vi "TLB Native Dynamic Events ver 0.08.vi"() -> ()   [LabVIEW 2018]
uses:
  Labview Training Phase 2/Enum Controls/States for Action Engine.ctl
  Type def/TLB event states.ctl
  Type def/TLB MHL States.ctl
  <vilib>/Studica/Studica Toolkit/Background/I2C Channel.ctl
  <vilib>/Studica/Studica Toolkit/NavX/NavX.lvlib
  <vilib>/myRIO/Common/Instrument Driver Framework/myRIO v1.0/AI/typedefs/AI Channels Enum.ctl
  <vilib>/myRIO/Common/Instrument Driver Framework/myRIO v1.0/AI/typedefs/AI Channels List.ctl
  Type def/Type def.ctl
  <vilib>/Studica/Studica Blackhawk/Blackhawk.lvlib
  <vilib>/Studica/Studica Toolkit/Background/Mxp Selection.ctl
  <vilib>/Studica/Studica Toolkit/Background/DIO Channel.ctl
  <vilib>/NI_Real-Time Target Support.lvlib
  <vilib>/ptbypt/NI_PtbyPt.lvlib
  <vilib>/addons/control/pid/NI_PID_pid.lvlib
  <vilib>/addons/control/pid/pid.llb/PID (DBL).vi
  Underlying VI's/Webcam FGV Low level ver/State control.ctl
  <vilib>/userdefined/High Color/IMAQdx.ctl
panel:
  out "Manual Zero Yaw":bool
  out "Displacement":T1
  out "Fused Heading":dbl
  in  "error in (no error)":errorcluster
  in  "RED LED State":enum16{"OFF", "ON", "BLINK"}(ring)
  in  "GREEN LED State":enum16{"OFF", "ON", "BLINK"}(ring)
  in  "Red LED":bool
  in  "Green LED":bool
  in  "NavX Zero Yaw":bool
  out "Input state":i8
  out "Waveform Chart 2":dbl(graph)
  out "Waveform Chart":dbl(graph)
  in  "STOP":bool
  out "DIO 0":bool
  out "DIO 1":bool
  out "Limit Switch Array":bool[](array[boolean])
  out "error out":errorcluster
  out "L/R average":fxp<+,64,64>
  out "Right Ultrasonic":fxp<+,64,16>
  out "Left Ultrasonic":fxp<+,64,16>
  out "Right IR Sensor":dbl
  out "Left IR Sensor":dbl
  out "Object detection count":T2
  out "Camera error":errorcluster
  in  "Servo Angle":u8(slide) scale=0.0..180.0
  in  "On/Off":bool
  out "Error":errorcluster
  out "element":T3
  out "Action Queue Items":i32
  out "State Logic Queue Items":i32
  out "Action Queues items":string[](array[string])=["Hardware reset", "Software reset", ""]
  out "State logic":T4=enum."Task 2"
  out "Action State":string
  out "Yaw":dbl
  # "TLB FRAMEWORK STATUS"
  # "Camera Status Loop"
  # "Test Programme written by Calvin Loke    Dated: 28 Aug 2019\nTest Programme revised by Dr Alex See   Dated 30 Aug 2019\n\nProgramme version:   TLB Native Dynamic Events ver 0.04b.vi"
  # "Problems now:\nYaw does not work when code is in last state mode\nSlow acceleration due to loop rate?"
  # "Motor Control Loop"
  # "NAVX Control Loop"
  # "Blackhawk status"
  # "Sensor data"
  # "System Health Status Update"
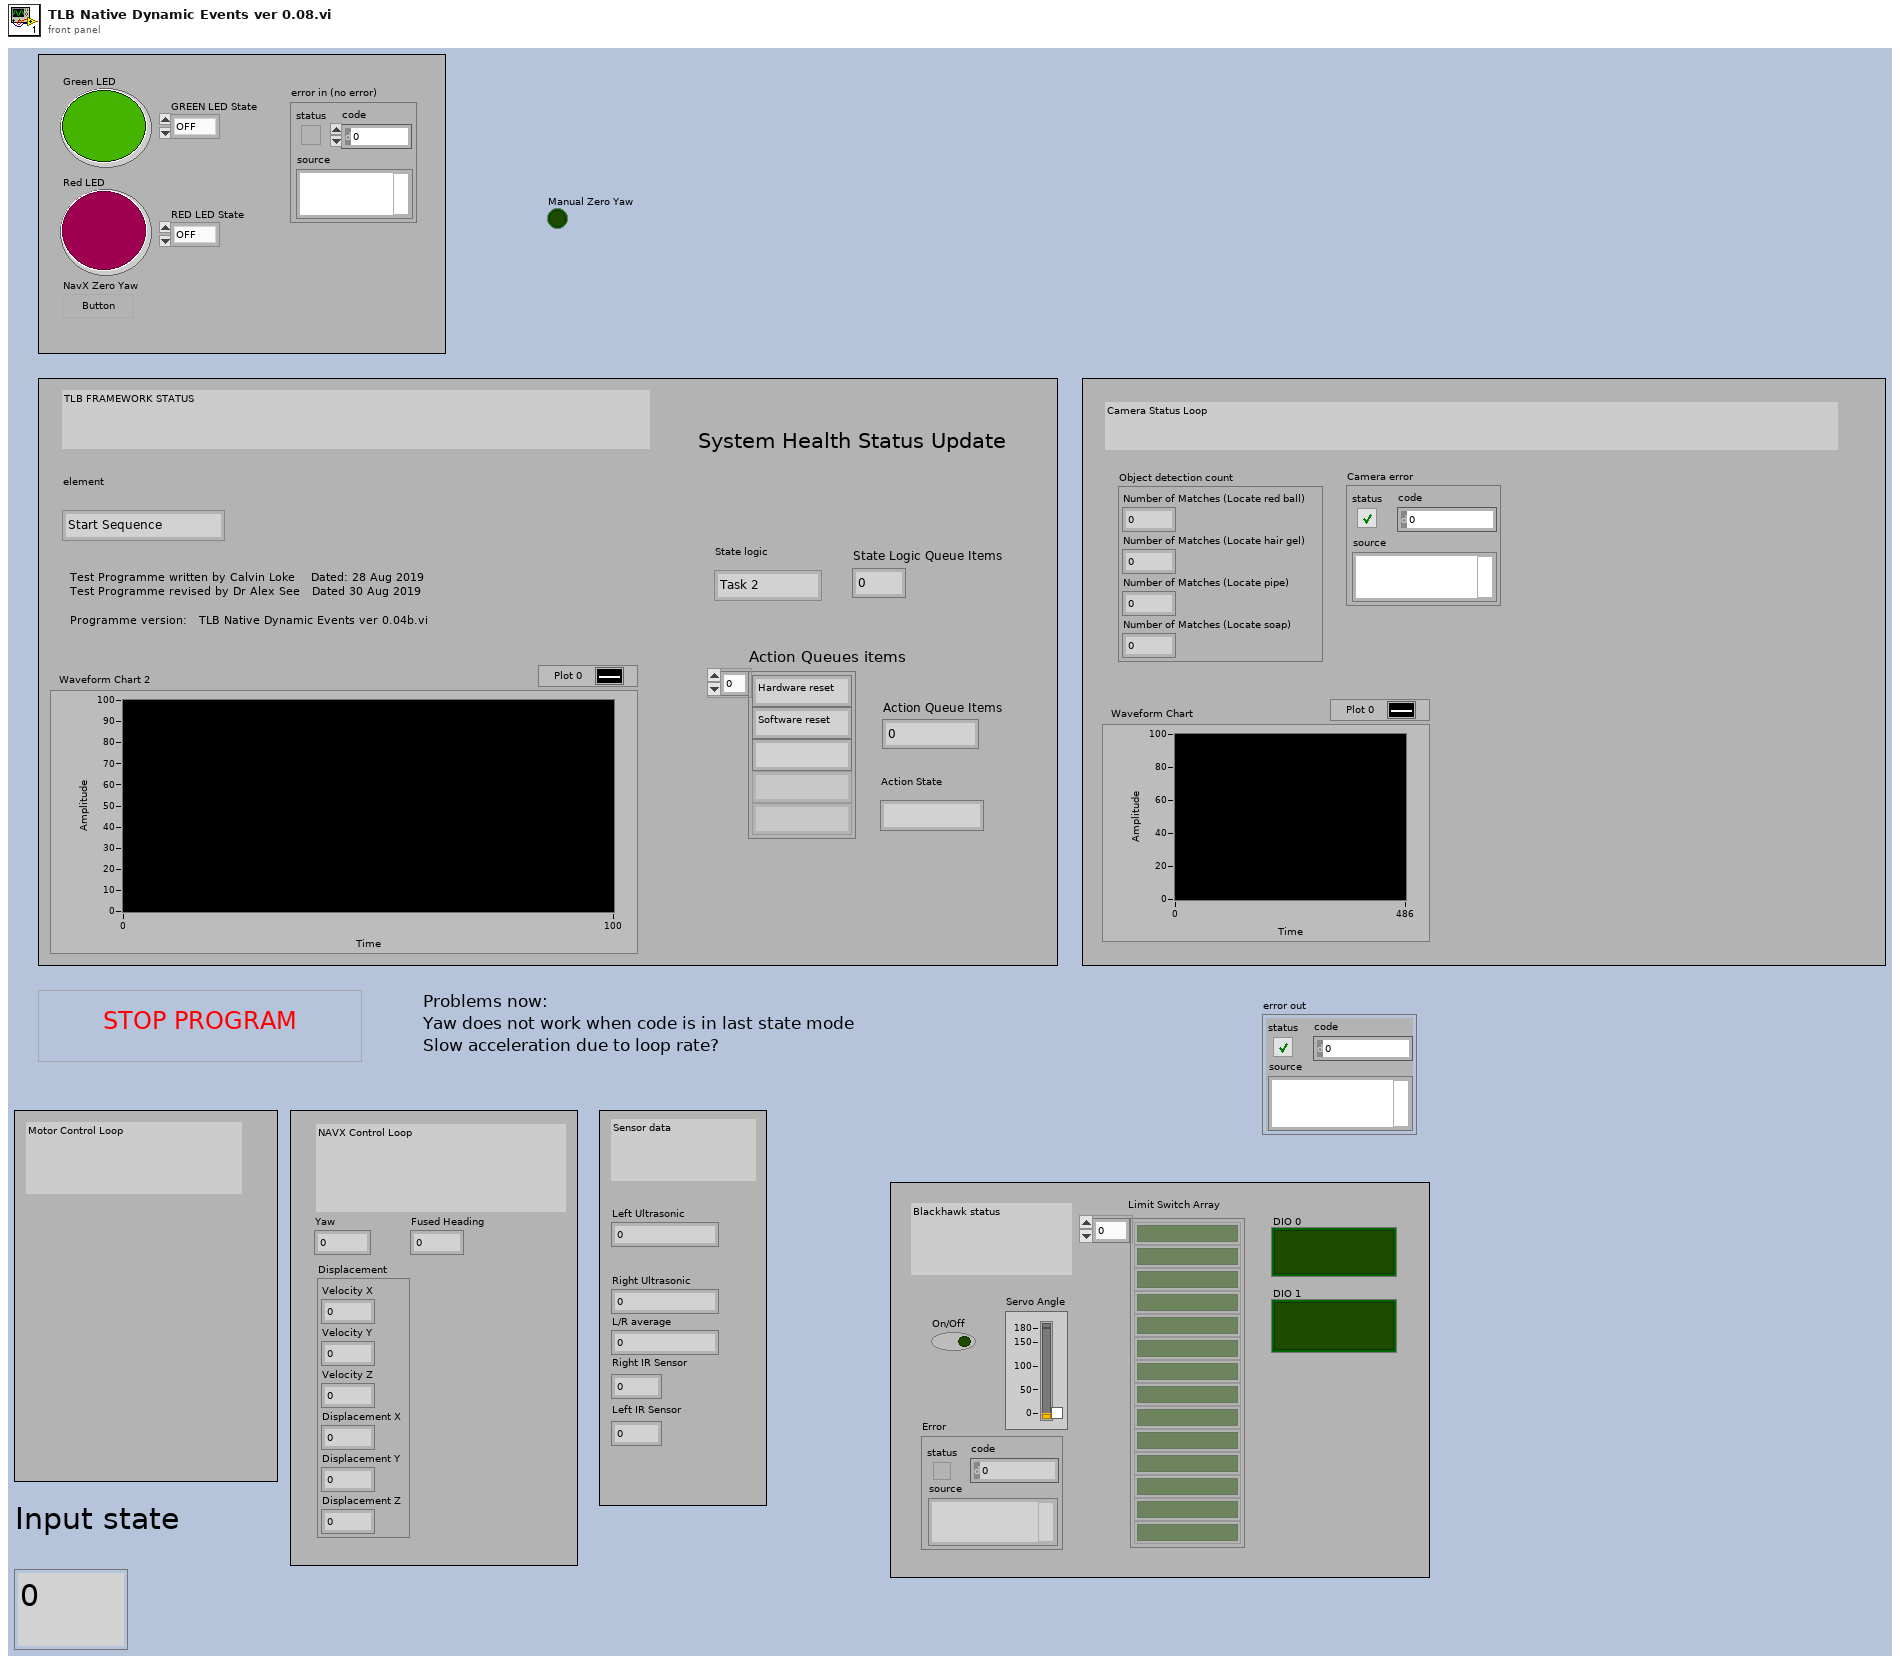
[diagram p1: front panel]
types:
  T1 = cluster{"Velocity X":dbl, "Velocity Y":dbl, "Velocity Z":dbl, "Displacement X":dbl, "Displacement Y":dbl, "Displacement Z":dbl}
  T2 = cluster{"Number of Matches (Locate red ball)":i32, "Number of Matches (Locate hair gel)":i32, "Number of Matches (Locate pipe)":i32, "Number of Matches (Locate soap)":i32}
  T3 = typedef "TLB event states.ctl" = enum16{"Start Sequence", "Exit", "Start Task 1", "Start Task 2", "Start Task 3", "Start Task 4", "Camera vision", "Wall follow mode", "Idle", "Start Drive Straight"}
  T4 = typedef "TLB MHL States.ctl" = enum16{"None", "Startup", "Idle", "Processing", "Shutdown", "Reset", "Task 1", "Task 2", "Task 3", "Task 4", "Task 4a", "Task 4b", "Task 4c", "Task 4d", "Task 4e", "Task 4f", "Task 4g", "Task 4h", "Acquire image", "Wall follow mode", "Autodrive", "Autodrive a"}
  T5 = typedef "States for Action Engine.ctl" = enum16{"Initialize", "Write", "Read"}
  T6 = typedef "DIO Channel.ctl" = enum16{"Not Connected", "A/DIO1", "A/DIO2", "A/DIO3", "A/DIO4", "A/DIO5", "A/DIO6", "A/DIO7", "A/DIO13", "B/DIO1", "B/DIO2", "B/DIO3", "B/DIO4", "B/DIO5", "B/DIO6", "B/DIO7", "B/DIO13", "C/DIO0", "C/DIO1", "C/DIO2", "C/DIO3", "C/DIO4", "C/DIO5", "C/DIO6", "C/DIO7"}
  T7 = typedef "Type def.ctl" = cluster{"Front Ultrasonic Obstruct":bool, "Left Ultrasonic Obstruct":bool, "Right Ultrasonic Obstruct ":bool}
  T8 = typedef "I2C Channel.ctl" = enum16{"Not Connected", "A", "B"}
  T9 = typedef "TLB MHL States.ctl" = enum16{"None", "Startup", "Idle", "Processing", "Shutdown", "Reset", "Task 1", "Task 2", "Task 3", "Task 4", "Task 4a", "Task 4b", "Task 4c", "Task 4d", "Task 4e", "Task 4f", "Task 4g", "Task 4h", "Acquire image", "Wall follow mode", "Drive Straight"}
  T10 = enum16{"LAST STATE", "STOP", "FORWARD", "BACKWARD", "LEFT", "RIGHT", "RCW", "ACW", "INIT", "RESET ENCODERS"}
  T11 = cluster{"proportional gain (Kc)":dbl, "integral time (Ti, min)":dbl, "derivative time (Td, min)":dbl}
  T12 = typedef "State control.ctl" = enum16{"Initialise", "Start camera", "Continuous Acquisition ", "Stop camera", "Dispose all"}
  T13 = typedef "IMAQdx.ctl" = refnum<k21>
  T14 = typedef "Mxp Selection.ctl" = enum16{"MXP A", "MXP B"}
  T15 = enum16{"DISTANCE READ", "STOP", "FORWARD", "BACKWARD", "LEFT", "RIGHT", "RCW", "ACW", "INIT", "RESET ENCODERS"}
  T16 = typedef "AI Channels List.ctl" = T17[]
  T17 = typedef "AI Channels Enum.ctl" = enum16{"Not Connected", "AudioIn/Left", "AudioIn/Right", "C/AI0", "C/AI1", "A/AI0", "A/AI1", "A/AI2", "A/AI3", "A/AI4", "A/AI5", "A/AI6", "A/AI7", "B/AI0", "B/AI1", "B/AI2", "B/AI3", "B/AI4", "B/AI5", "B/AI6", "B/AI7", "AI/AI0", "AI/AI1", "AI/AI2", "AI/AI3", "A/AI0 (DIFF)", "A/AI1 (DIFF)", "A/AI2 (DIFF)", "A/AI3 (DIFF)", "B/AI0 (DIFF)", "B/AI1 (DIFF)", "B/AI2 (DIFF)", "B/AI3 (DIFF)"}
  T18 = cluster{"DIO Channel":T6, "FPGA VI Reference Out":refnum<k20>}
  T19 = typedef "Analog Scaling Constants List.ctl" = T20[]
  T20 = typedef "Analog Scaling Constants.ctl" = cluster{"LSB Weight (Volts)":dbl, "Offset (Volts)":dbl, "Signed?":bool}
  T21 = cluster{"Scale Constants Array":T19, "FPGA Reference Out":refnum<k20>, "AI Channel":T16}
  T22 = cluster{"I2C Channel":T8, "FPGA VI Reference Out":refnum<k20>}
  T23 = typedef "NI_Real-Time Target Support.lvlib/RT CPU Load.ctl" = cluster{"Total (%)":dbl, "Time Critical (%)":dbl, "Timed Structures (%)":dbl, "High (%)":dbl, "Above Normal (%)":dbl, "Normal (%)":dbl, "Background (%)":dbl, "Idle (%)":dbl, "ISR (%)":dbl}
  T24 = cluster{"CPU loads[0]":T23, "CPU loads[1]":T23, "CPU loads[2]":T23, "CPU loads[3]":T23, "CPU loads[4]":T23, "CPU loads[5]":T23, "CPU loads[6]":T23, "CPU loads[7]":T23, "CPU loads[8]":T23}
  T25 = cluster{"I2C Ref Out":cluster{"I2C Channel":T8, "FPGA VI Reference Out":refnum<k20>}, "Connected":bool, "Slave Address (7-bit)":u8, "Registry":u8[]}
  T26 = cluster{"Yaw":dbl, "Roll":dbl, "Pitch":dbl, "Heading":dbl, "Fused Heading":dbl}
  T27 = typedef "IMAQ Image.ctl" = refnum<image>
  T28 = cluster{cluster{"xSpeed":dbl, "ySpeed":dbl, "wSpeed":dbl}, cluster{"xDistance":dbl, "yDistance":dbl, "wDistance":dbl}}
  T29 = cluster{"xDistance":dbl, "yDistance":dbl, "wDistance":dbl}
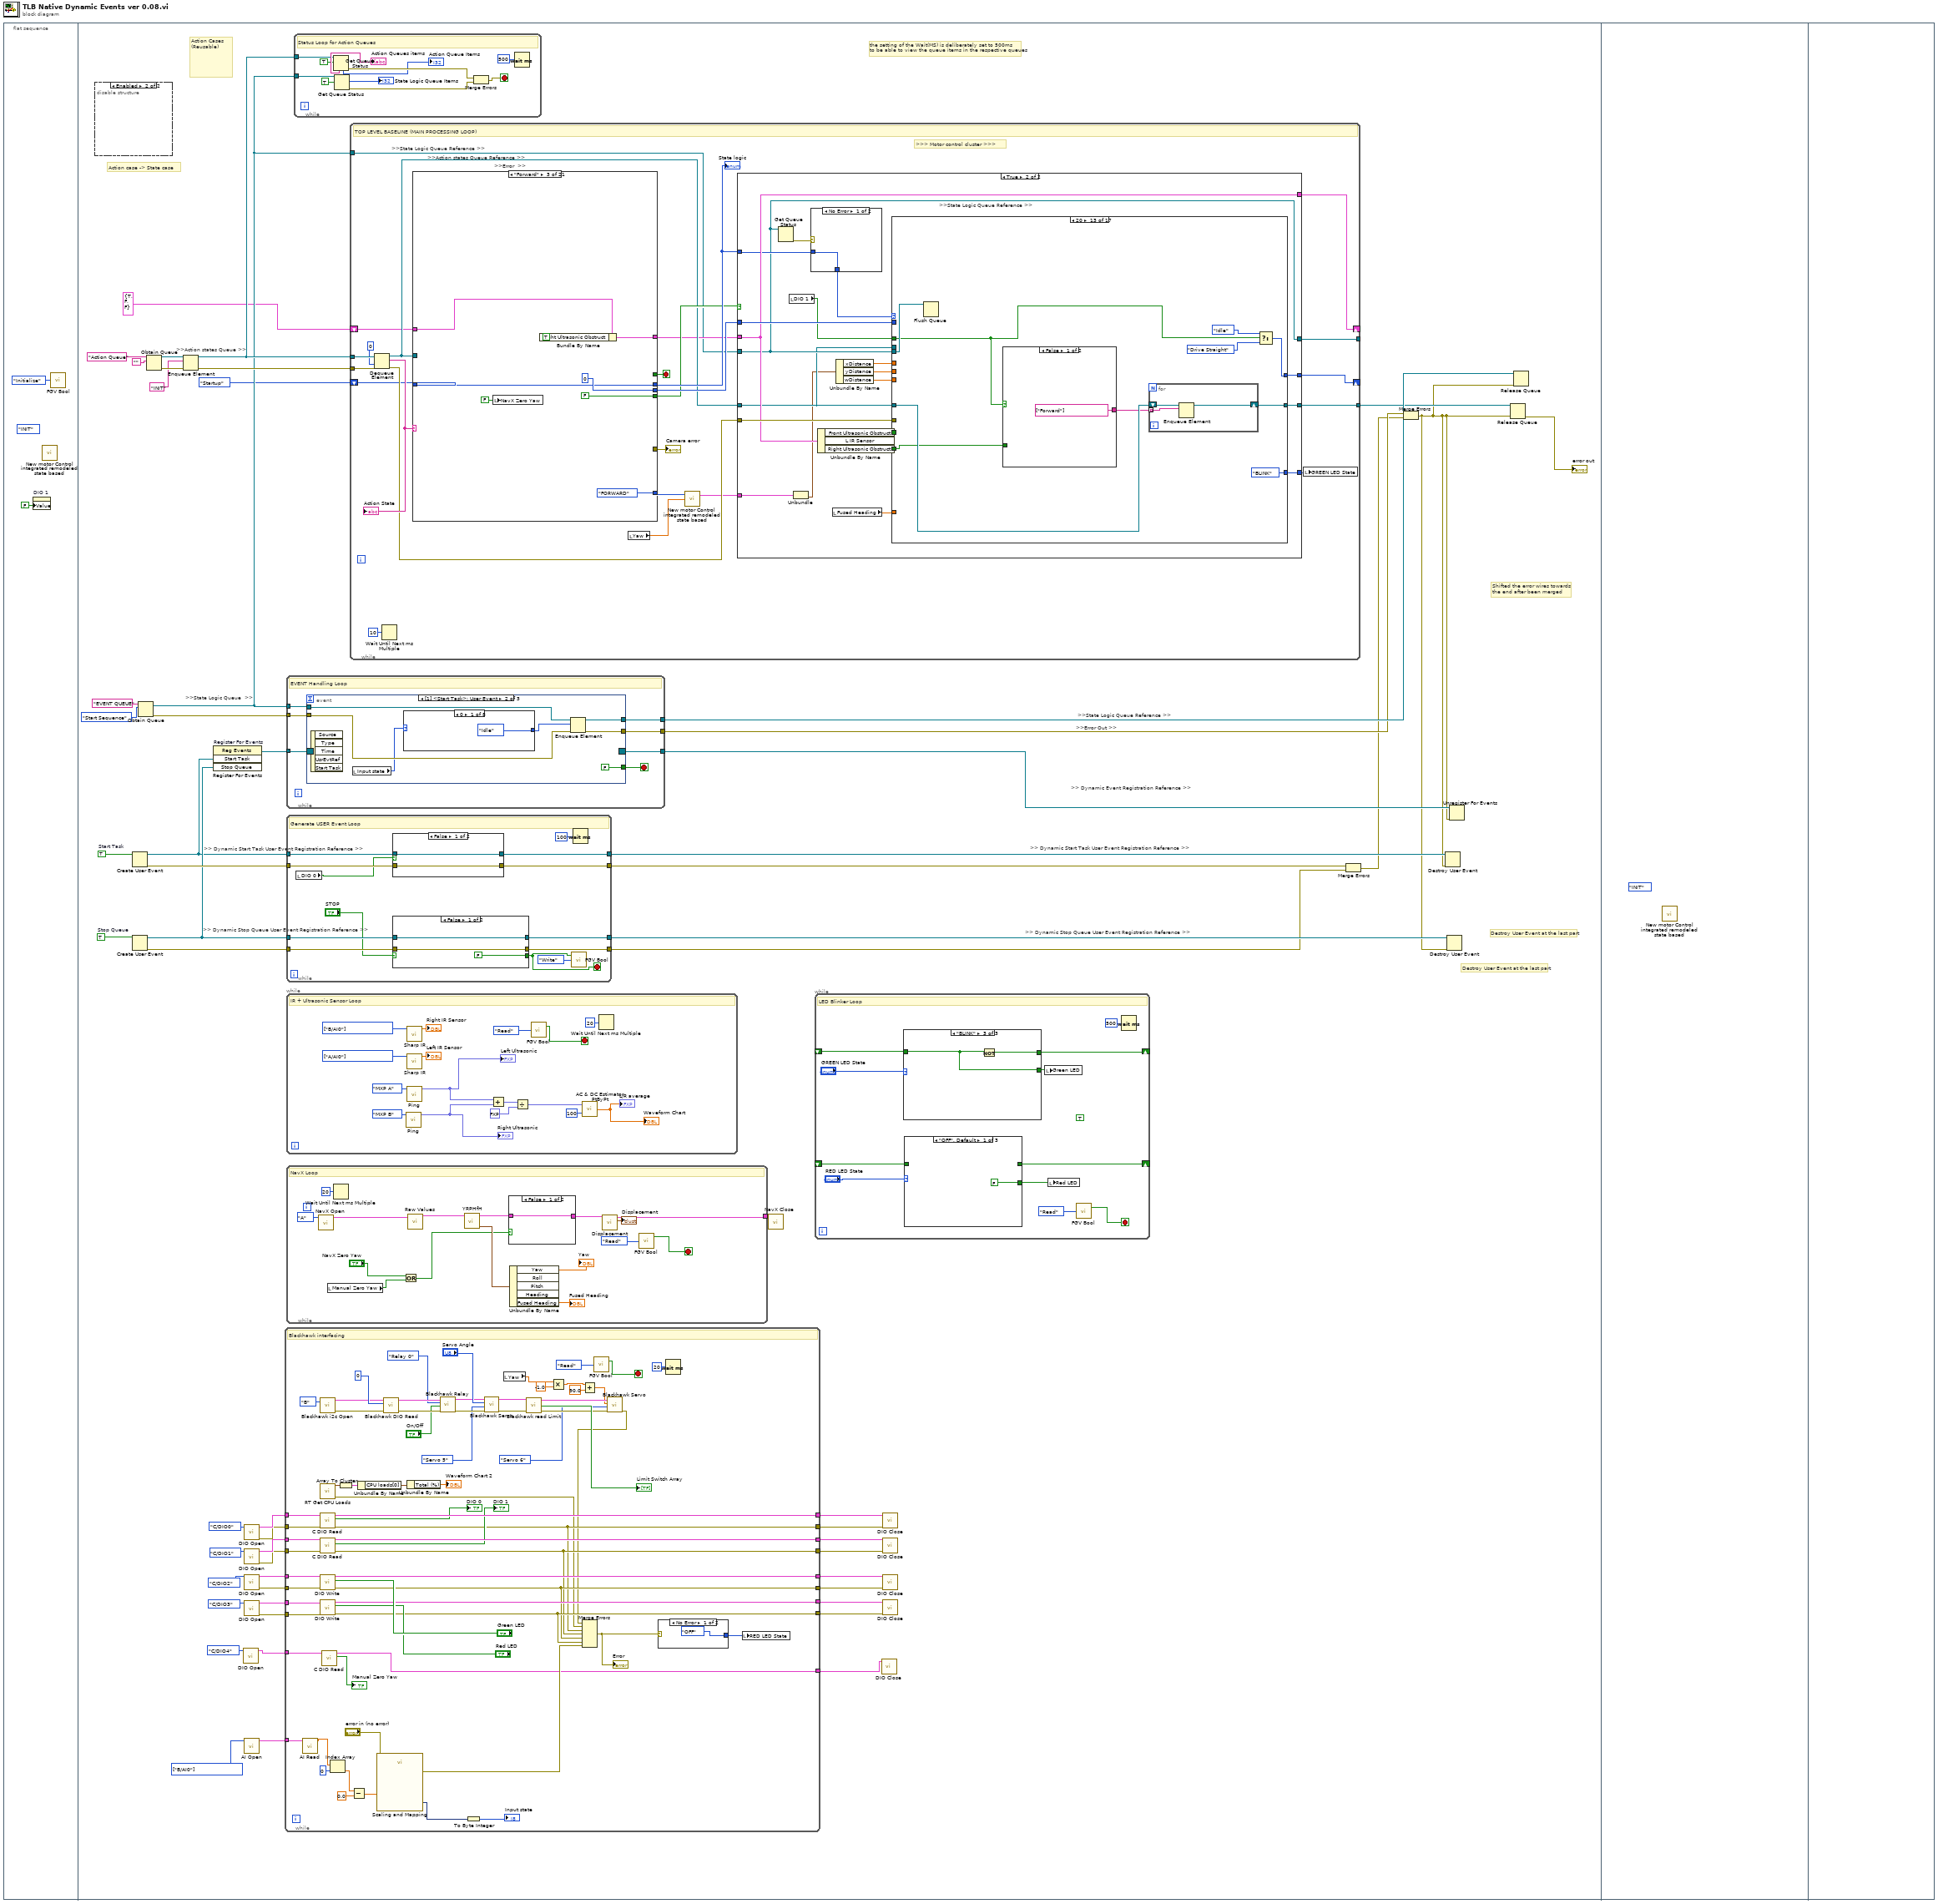
[diagram p0: block diagram]
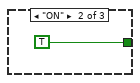
[diagram p2: hidden frame]
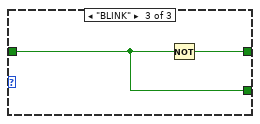
[diagram p3: hidden frame]
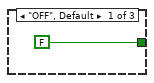
[diagram p4: hidden frame]
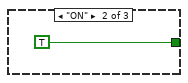
[diagram p5: hidden frame]
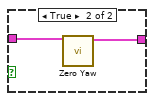
[diagram p6: hidden frame]
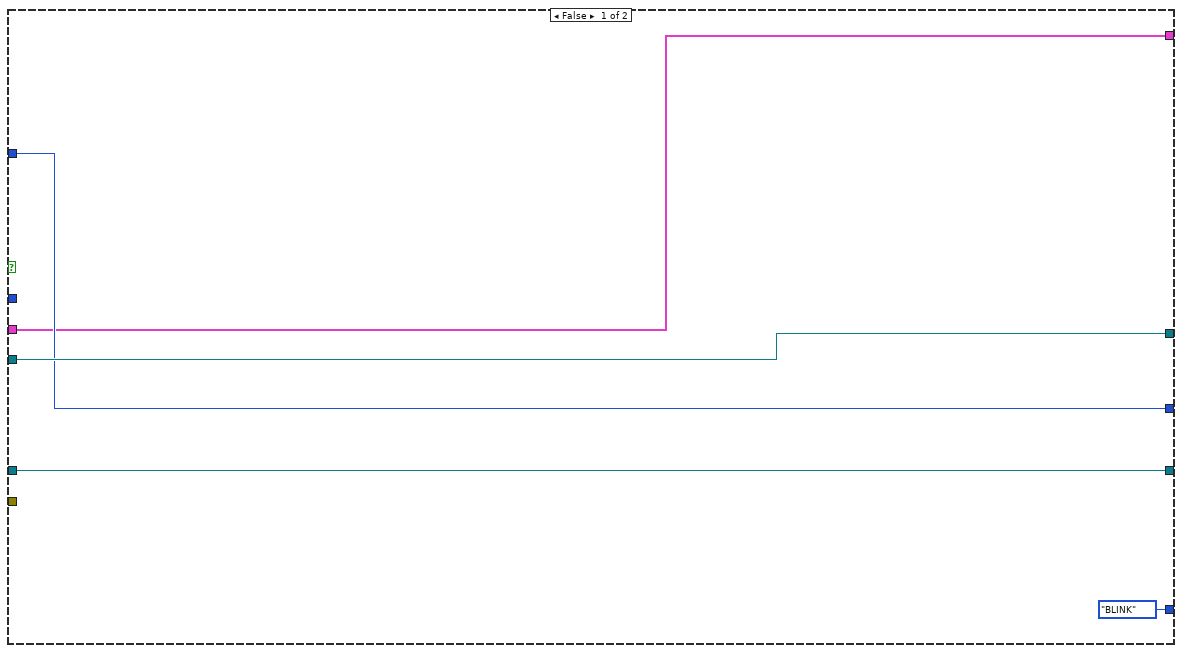
[diagram p7: hidden frame]
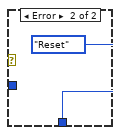
[diagram p8: hidden frame]
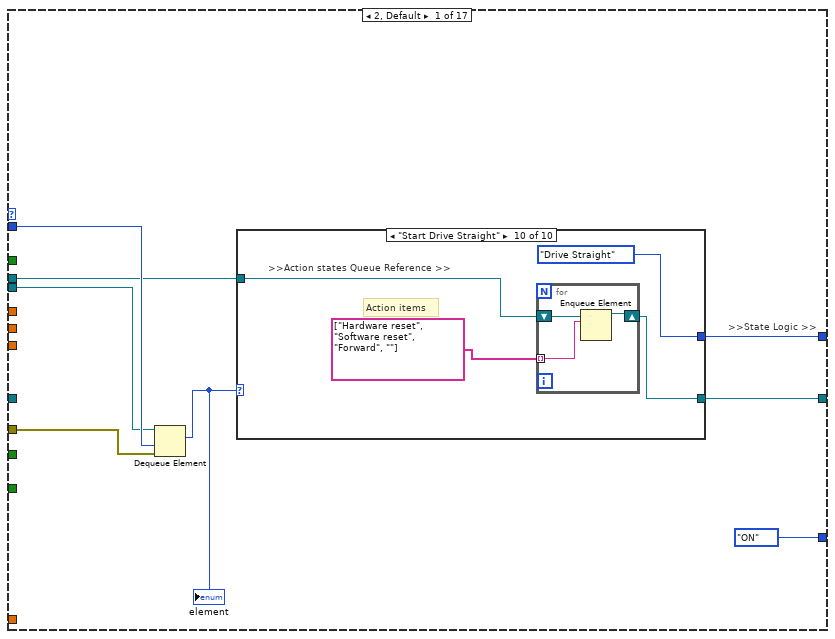
[diagram p9: hidden frame]
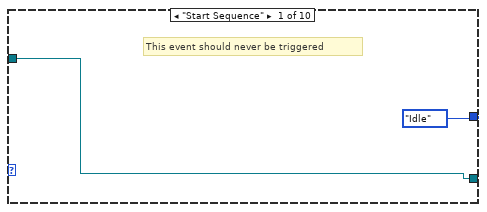
[diagram p10: hidden frame]
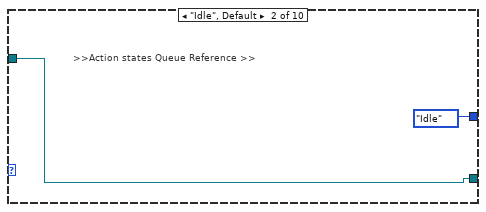
[diagram p11: hidden frame]
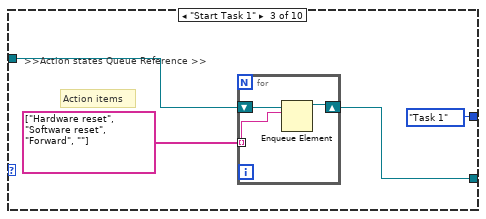
[diagram p12: hidden frame]
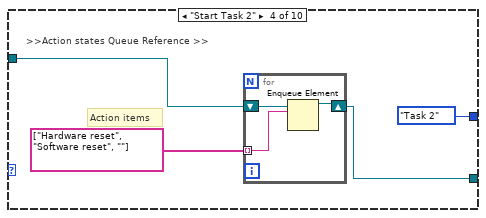
[diagram p13: hidden frame]
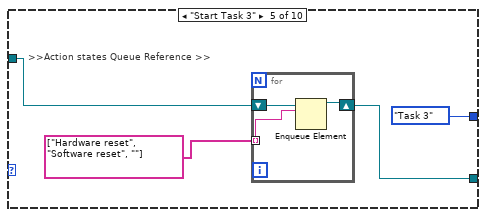
[diagram p14: hidden frame]
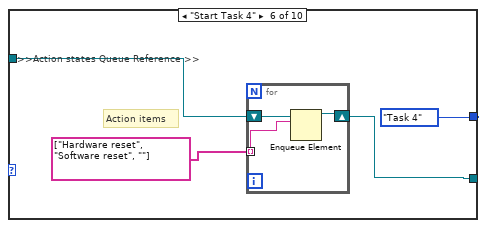
[diagram p15: hidden frame]
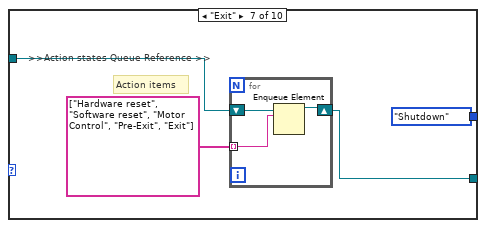
[diagram p16: hidden frame]
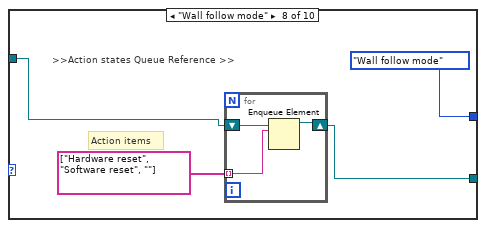
[diagram p17: hidden frame]
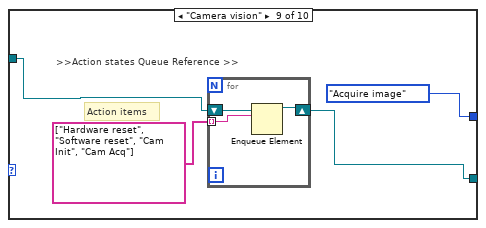
[diagram p18: hidden frame]
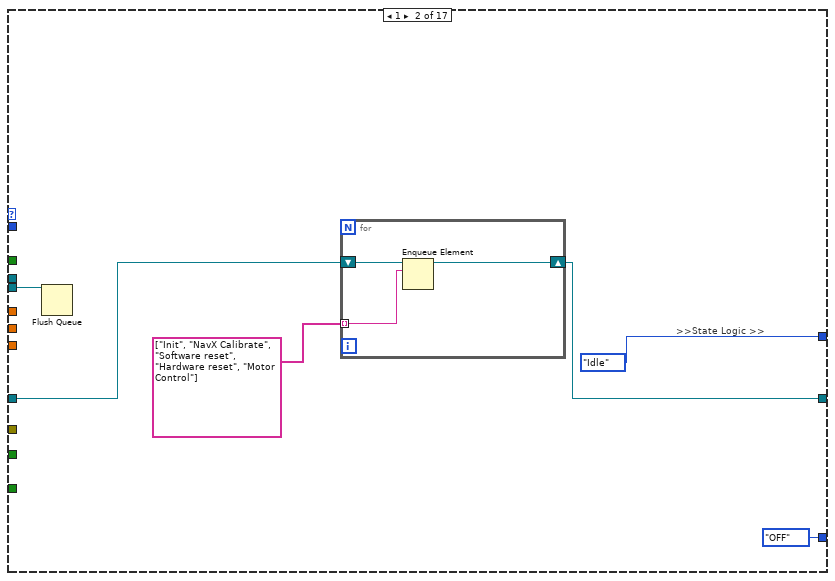
[diagram p19: hidden frame]
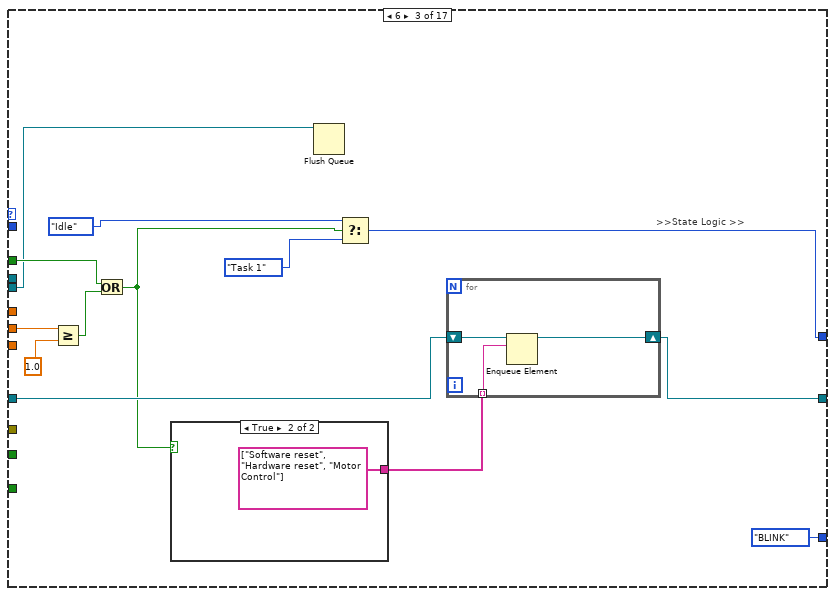
[diagram p20: hidden frame]
diagram:
  n1 = flat-sequence {
    frame #0 {
      (unwired) T15."INIT" ("States")
      n2 = property on="DIO 1" class="Bool (strict)"("Value"=FALSE ("DIO 1")) -> ()  [unwired: 2 in, 2 out]
      n3 = call "New motor Control integrated remodeled state based.vi"() -> ()  [unwired: 3 in, 2 out]
      n4 = call "FGV Bool.vi"("Init/Read/Write State"=States_for_Action_Engine."Initialize") -> ()  [unwired: 2 in, 2 out]
    }
    frame #1 {
      w11 = T16 [enum."B/AI0"] items=["Not Connected", "AudioIn/Left", "AudioIn/Right", "C/AI0", "C/AI1", "A/AI0", "A/AI1", "A/AI2", "A/AI3", "A/AI4", "A/AI5", "A/AI6", "A/AI7", "B/AI0", "B/AI1", "B/AI2", "B/AI3", "B/AI4", "B/AI5", "B/AI6", "B/AI7", "AI/AI0", "AI/AI1", "AI/AI2", "AI/AI3", "A/AI0 (DIFF)", "A/AI1 (DIFF)", "A/AI2 (DIFF)", "A/AI3 (DIFF)", "B/AI0 (DIFF)", "B/AI1 (DIFF)", "B/AI2 (DIFF)", "B/AI3 (DIFF)"] ("AI Channel")
      w59 = TRUE  # Stop Queue
      w58 = TRUE  # Start Task
      # "Action case -> State case"
      # "the setting of the Wait(MS) is deliberately set to 500ms\nto be able to view the queue items in the respective queues"
      # "Action Cases\n(Reusable)"
      # ">>Error Out >>"
      # ">> Dynamic Stop Queue User Event Registration Reference >>"
      # ">> Dynamic Start Task User Event Registration Reference >>"
      # ">> Dynamic Stop Queue User Event Registration Reference >>"
      # ">> Dynamic Start Task User Event Registration Reference >>"
      # ">> Dynamic Event Registration Reference >>"
      # ">>Action states Queue >>"
      # ">>State Logic Queue  >>"
      # ">>State Logic Queue Reference >>"
      # "Destroy User Event at the last part"
      # "Destroy User Event at the last part"
      # "Shifted the error wires towards\nthe end after been merged"
      n5 = disable-structure shown="Enabled" {
        frame Disabled {
          (unwired) variant
          (unwired) TRUE
          n6 = Variant To Data(type="") -> ()  [unwired: 2 in, 2 out]
        }
        frame Enabled {
        }
      }
      n7 = Create User Event(user event datatype=w58) -> (user event=w50:refnum<user-event>, error out=w55:errorcluster)  [unwired: 1 in]
      n8 = Create User Event(user event datatype=w59) -> (user event=w51:refnum<user-event>, error out=w54:errorcluster)  [unwired: 1 in]
      n9 = Obtain Queue(name (unnamed)="EVENT QUEUE", element data type=TLB_event_states."Start Sequence" ("Enum")) -> (queue out=w35:refnum<queue>, error out=w41:errorcluster)  [unwired: 3 in, 1 out]
      n10 = Obtain Queue(name (unnamed)="Action Queue", element data type="") -> (queue out=w44:refnum<queue>, error out=w40:errorcluster)  [unwired: 3 in, 1 out]
      n11 = Enqueue Element(queue=w44, element="INIT", error in (no error)=w40) -> (queue out=w36:refnum<queue>, error out=w39:errorcluster)  [unwired: 1 in, 1 out]
      n12 = register-events "Register For Events"(w50, w51) -> (reference out=w49:refnum<event-registration>)  [unwired: 2 in, 1 out]
      n13 = call <vilib>:"DIO Open.vi"("DIO Channel"=DIO_Channel."C/DIO4") -> ("DIO Info Out"=w5:T18)  [unwired: 9 in, 1 out]
      n14 = call <vilib>:"DIO Open.vi"("DIO Channel"=DIO_Channel."C/DIO0") -> ("error out"=w21:errorcluster, "DIO Info Out"=w27:T18)  [unwired: 9 in]
      n15 = call <vilib>:"DIO Open.vi"("DIO Channel"=DIO_Channel."C/DIO1") -> ("error out"=w19:errorcluster, "DIO Info Out"=w23:T18)  [unwired: 9 in]
      n16 = call <vilib>:"DIO Open.vi"("DIO Channel"=DIO_Channel."C/DIO2") -> ("error out"=w9:errorcluster, "DIO Info Out"=w15:T18)  [unwired: 9 in]
      n17 = call <vilib>:"DIO Open.vi"("DIO Channel"=DIO_Channel."C/DIO3") -> ("error out"=w7:errorcluster, "DIO Info Out"=w14:T18)  [unwired: 9 in]
      n18 = call <vilib>:"AI Open.vi"("AI Channel"=w11) -> ("Analog Info"=w10:T21)  [unwired: 9 in, 1 out]
      n19 = while {
        tunnel: w27 -> [w713]
        tunnel: [w712] -> w26
        tunnel: w23 -> [w711]
        tunnel: [w710] -> w22
        tunnel: w21 -> [w709]
        tunnel: [w678] -> w20
        tunnel: w19 -> [w708]
        tunnel: [w679] -> w18
        tunnel: w15 -> [w702]
        tunnel: w14 -> [w701]
        tunnel: [w698] -> w13
        tunnel: [w697] -> w12
        tunnel: w10 -> [w696]
        tunnel: w9 -> [w689]
        tunnel: [w680] -> w8
        tunnel: w7 -> [w688]
        tunnel: [w681] -> w6
        tunnel: w5 -> [w669]
        tunnel: [w668] -> w3
        stop <- w726 stop-if-true
        # "Blackhawk interfacing"
        n20 = call <vilib>:"AI Read.vi"("Analog Info"=w696) -> ("Array"=w692:dbl[])  [unwired: 9 in, 1 out]
        n21 = call <vilib>:"Blackhawk i2c Open.vi"("I2C Channel"=I2C_Channel."B") -> ("I2C Ref Out"=w704:T22, "error out"=w703:errorcluster)  [unwired: 2 in]
        n22 = call <vilib>:"RT Get CPU Loads.vi"() -> ("error out"=w677:errorcluster, "CPU loads"=w683:T23[])  [unwired: 10 in]
        n23 = call <vilib>:"C DIO Read.vi"("error in (no error)"=w709, "DIO Info In in"=w713) -> ("error out"=w678:errorcluster, "IN"=→"DIO 0":bool, "DIO Info In out"=w712:T18)  [unwired: 7 in]
        n24 = call <vilib>:"C DIO Read.vi"("error in (no error)"=w708, "DIO Info In in"=w711) -> ("error out"=w679:errorcluster, "IN"=→"DIO 1":bool, "DIO Info In out"=w710:T18)  [unwired: 7 in]
        n25 = call <vilib>:"DIO Write.vi"("error in (no error)"=w689, "Input"="Green LED", "DIO Info In"=w702) -> ("error out"=w680:errorcluster, "DIO Info Out"=w698:T18)  [unwired: 7 in]
        n26 = call <vilib>:"DIO Write.vi"("error in (no error)"=w688, "Input"="Red LED", "DIO Info In"=w701) -> ("error out"=w681:errorcluster, "DIO Info Out"=w697:T18)  [unwired: 7 in]
        n27 = call <vilib>:"C DIO Read.vi"("DIO Info In in"=w669) -> ("IN"=→"Manual Zero Yaw":bool, "DIO Info In out"=w668:T18)  [unwired: 8 in, 1 out]
        n28 = Index Array(array=w692, index=0) -> (element=w694:dbl)
        n29 = Array To Cluster(array=w683) -> (cluster=w684:T24)
        n30 = Subtract(x=w694, y=0.0) -> (x-y=w695:dbl)
        n31 = Unbundle By Name(w684) -> ("CPU loads[0]"=w685:T23)
        n32 = call "Scaling and Mapping"("error in (no error)"="error in (no error)", "Signals"=w695) -> ("error out"=w682:errorcluster, "Scaled Signals"=w690:dynamicdata)  [unwired: 8 in]
        n33 = call <vilib>:"Blackhawk DIO Read.vi"("I2C Ref In"=w704, "PIN"=u8 0, "error in (no error)"=w703) -> ("I2C Ref Out"=w724:T22, "error out"=w725:errorcluster)  [unwired: 3 in, 1 out]
        n34 = Unbundle By Name(w685) -> ("Total (%)"=→"Waveform Chart 2":dbl)
        n35 = call <vilib>:"Blackhawk Relay.vi"("error in (no error)"=w725, "On/Off"="On/Off", "Relay"=enum8{"Relay 0", "Relay 1", "Relay 2"}."Relay 0", "I2C Ref In"=w724) -> ("error out"=w721:errorcluster, "I2C Ref Out"=w718:T22)  [unwired: 6 in]
        n36 = To Byte Integer(number=w690) -> (8bit integer=→"Input state":i8)
        n37 = call <vilib>:"Blackhawk Servo.vi"("error in (no error)"=w721, "Servo Select"=enum16{"Servo 5", "Servo 6"}."Servo 5", "Servo Angle"="Servo Angle", "I2C Ref In"=w718) -> ("error out"=w716:errorcluster, "I2C Ref Out"=w715:T22)  [unwired: 6 in]
        n38 = local read "Yaw"() -> (w663:dbl)
        n39 = call <vilib>:"Blackhawk read Limit.vi"("error in (no error)"=w716, "I2C Ref In"=w715) -> ("error out"=w673:errorcluster, "Limit Switch Array"=→"Limit Switch Array":bool[], "I2C Ref Out"=w671:T22)  [unwired: 1 in]
        n40 = Multiply(x=w663, y=-1.0) -> (x*y=w664:dbl)
        n41 = Add(x=w664, y=90.0) -> (x+y=w665:dbl)
        n42 = call "FGV Bool.vi"("Init/Read/Write State"=States_for_Action_Engine."Read") -> ("Output node"=w726:bool)  [unwired: 2 in, 1 out]
        n43 = call <vilib>:"Blackhawk Servo.vi"("error in (no error)"=w673, "Servo Select"=enum16{"Servo 5", "Servo 6"}."Servo 6", "Servo Angle"=w665, "I2C Ref In"=w671) -> ("error out"=w672:errorcluster)  [unwired: 6 in, 1 out]
        n44 = Merge Errors(w672, w677, w678, w679, w680, w681, w682) -> (w676:errorcluster)
        "Error" <- w676
        n45 = case shown="No Error" w676 {
          tunnel: [enum16{"OFF", "ON", "BLINK"}."OFF" ("RED LED State") enum16{"OFF", "ON", "BLINK"}."BLINK" ("RED LED State")] -> w687
          frame No Error {
          }
          frame Error {
          }
        }
        n46 = Wait (ms)(milliseconds to wait=u32 20) -> ()  [unwired: 1 out]
        n47 = local write "RED LED State"(w687) -> ()
      }
      n48 = while {
        tunnel: w49 -> [w606]
        tunnel: [w605] -> w48
        tunnel: w35 -> [w603]
        tunnel: [w602] -> w47
        tunnel: w41 -> [w601]
        tunnel: [w600] -> w38
        stop <- w604 stop-if-true
        # "EVENT Handling Loop"
        n49 = event shown="[1] <Start Task>: User Event" {
          selector: w606 -> [_ _ _]
          dyn-events: [_ _ _] -> w605
          timeout: _ -> [_ _ _]
          tunnel: [FALSE FALSE w633] -> w604
          tunnel: w603 -> [w611 w618 w631]
          tunnel: [w610 w617 w632] -> w602
          tunnel: w601 -> [w608 w616 w629]
          tunnel: [w607 w615 w628] -> w600
          event Timeout {
            n50 = event-data() -> ()  [unwired: 1 in, 3 out]
            n51 = Enqueue Element(queue=w611, element=TLB_event_states."Idle" ("Enum"), error in (no error)=w608) -> (queue out=w610:refnum<queue>, error out=w607:errorcluster)  [unwired: 1 in, 1 out]
          }
          event User Event {
            n52 = event-data() -> ()  [unwired: 1 in, 5 out]
            n53 = local read "Input state"() -> (w614:i8)
            n54 = case shown="0" w614 {
              tunnel: [TLB_event_states."Idle" ("Enum") TLB_event_states."Start Task 1" ("Enum") TLB_event_states."Start Task 2" ("Enum") TLB_event_states."Start Task 3" ("Enum") TLB_event_states."Start Task 4" ("Enum") TLB_event_states."Wall follow mode" ("Enum") TLB_event_states."Camera vision" ("Enum") TLB_event_states."Start Drive Straight" ("Enum")] -> w613
              frame 0 {
              }
              frame 1 {
              }
              frame 2 {
              }
              frame 3, Default {
              }
              frame 4 {
              }
              frame 5 {
              }
              frame 6 {
              }
              frame 7 {
              }
            }
            n55 = Enqueue Element(queue=w618, element=w613, error in (no error)=w616) -> (queue out=w617:refnum<queue>, error out=w615:errorcluster)  [unwired: 1 in, 1 out]
          }
          event User Event {
            n56 = event-data() -> ("Stop Queue"=w633:bool)  [unwired: 1 in, 4 out]
            n57 = Enqueue Element At Opposite End(queue=w631, element=TLB_event_states."Exit" ("Enum"), error in (no error)=w629) -> (queue out=w632:refnum<queue>, error out=w628:errorcluster)  [unwired: 1 in, 1 out]
          }
        }
      }
      n58 = while {
        tunnel: w50 -> [w645]
        tunnel: w51 -> [w644]
        tunnel: [w643] -> w57
        tunnel: [w642] -> w56
        tunnel: w55 -> [w641]
        tunnel: [w640] -> w53
        tunnel: w54 -> [w639]
        tunnel: [w638] -> w52
        stop <- w636 stop-if-true
        # "Generate USER Event Loop"
        n59 = local read "DIO 0"() -> (w635:bool)
        n60 = case shown="False" w635 {
          selector: w635 -> [_ w657]
          tunnel: w645 -> [w656 w661]
          tunnel: [w656 w660] -> w642
          tunnel: w641 -> [w655 w659]
          tunnel: [w655 w658] -> w640
          frame False {
          }
          frame True {
            n61 = Generate User Event(user event=w661, event data cluster=w657, error in=w659) -> (user event out=w660:refnum<user-event>, error out=w658:errorcluster)  [unwired: 1 in]
          }
        }
        n62 = case shown="False" "STOP" {
          selector: "STOP" -> [_ w650]
          tunnel: w644 -> [w649 w654]
          tunnel: [w649 w653] -> w643
          tunnel: w639 -> [w648 w652]
          tunnel: [w648 w651] -> w638
          tunnel: [FALSE w650] -> w636
          frame False {
          }
          frame True {
            n63 = Generate User Event(user event=w654, event data cluster=w650, error in=w652) -> (user event out=w653:refnum<user-event>, error out=w651:errorcluster)  [unwired: 1 in]
          }
        }
        n64 = call "FGV Bool.vi"("Init/Read/Write State"=States_for_Action_Engine."Write", "Input Node"=w636) -> ()  [unwired: 1 in, 2 out]
        n65 = Wait (ms)(milliseconds to wait=u32 100) -> ()  [unwired: 1 out]
      }
      n66 = while {
        stop <- w582 stop-if-true
        w587 = T16 [enum."A/AI0"] items=["Not Connected", "AudioIn/Left", "AudioIn/Right", "C/AI0", "C/AI1", "A/AI0", "A/AI1", "A/AI2", "A/AI3", "A/AI4", "A/AI5", "A/AI6", "A/AI7", "B/AI0", "B/AI1", "B/AI2", "B/AI3", "B/AI4", "B/AI5", "B/AI6", "B/AI7", "AI/AI0", "AI/AI1", "AI/AI2", "AI/AI3", "A/AI0 (DIFF)", "A/AI1 (DIFF)", "A/AI2 (DIFF)", "A/AI3 (DIFF)", "B/AI0 (DIFF)", "B/AI1 (DIFF)", "B/AI2 (DIFF)", "B/AI3 (DIFF)"] ("AI Channel")
        w588 = T16 [enum."B/AI0"] items=["Not Connected", "AudioIn/Left", "AudioIn/Right", "C/AI0", "C/AI1", "A/AI0", "A/AI1", "A/AI2", "A/AI3", "A/AI4", "A/AI5", "A/AI6", "A/AI7", "B/AI0", "B/AI1", "B/AI2", "B/AI3", "B/AI4", "B/AI5", "B/AI6", "B/AI7", "AI/AI0", "AI/AI1", "AI/AI2", "AI/AI3", "A/AI0 (DIFF)", "A/AI1 (DIFF)", "A/AI2 (DIFF)", "A/AI3 (DIFF)", "B/AI0 (DIFF)", "B/AI1 (DIFF)", "B/AI2 (DIFF)", "B/AI3 (DIFF)"] ("AI Channel")
        # "IR + Ultrasonic Sensor Loop"
        n67 = call <vilib>:"Ping.vi"("Mxp Side"=Mxp_Selection."MXP B") -> ("CM"=w576:fxp<+,64,16>)  [unwired: 8 in, 2 out]
        "Right Ultrasonic" <- w576
        n68 = call <vilib>:"Ping.vi"("Mxp Side"=Mxp_Selection."MXP A") -> ("CM"=w577:fxp<+,64,16>)  [unwired: 8 in, 2 out]
        "Left Ultrasonic" <- w577
        n69 = call <vilib>:"Sharp IR.vi"("AI Channel"=w588) -> ("Sharp IR Distance"=→"Right IR Sensor":dbl)  [unwired: 8 in, 2 out]
        n70 = call <vilib>:"Sharp IR.vi"("AI Channel"=w587) -> ("Sharp IR Distance"=→"Left IR Sensor":dbl)  [unwired: 8 in, 2 out]
        n71 = Add(x=w577, y=w576) -> (x+y=w579:fxp<+,64,17>)
        n72 = Divide(x=w579, y=fxp<+,64,17> 2.0) -> (x/y=w575:fxp<+,64,64>)
        n73 = call "FGV Bool.vi"("Init/Read/Write State"=States_for_Action_Engine."Read") -> ("Output node"=w582:bool)  [unwired: 2 in, 1 out]
        n74 = call <vilib>:"AC & DC Estimator PtByPt.vi"("signal"=w575, "sample length"=100) -> ("DC estimate (V)"=→"L/R average" →"Waveform Chart":dbl)  [unwired: 1 in, 2 out]
        n75 = Wait Until Next ms Multiple(millisecond multiple=u32 20) -> ()  [unwired: 1 out]
      }
      n76 = while {
        tunnel: [w85] -> w28
        stop <- w93 stop-if-true
        # "NavX Loop"
        n77 = call <vilib>:"NavX Open.vi"("I2C Channel"=I2C_Channel."A") -> ("NavX Info"=w87:T25)  [unwired: 9 in, 1 out]
        n78 = local read "Manual Zero Yaw"() -> (w81:bool)
        n79 = Wait Until Next ms Multiple(millisecond multiple=u32 20) -> ()  [unwired: 1 out]
        n80 = Or(x="NavX Zero Yaw", y=w81) -> (x .or. y?=w82:bool)
        n81 = call <vilib>:"Raw Values.vi"("NavX Info In"=w87) -> ("NavX Info Out"=w90:T25)  [unwired: 8 in, 1 out]
        n82 = call <vilib>:"YRPHfH.vi"("NavX Info In"=w90) -> ("YRPHfH"=w91:T26, "NavX Info Out"=w89:T25)  [unwired: 3 in]
        n83 = case shown="False" w82 {
          tunnel: [w95 w97] -> w86
          tunnel: w89 -> [w95 w96]
          frame False {
          }
          frame True {
            n84 = call <vilib>:"Zero Yaw.vi"("NavX Info In"=w96) -> ("NavX Info Out"=w97:T25)  [unwired: 10 in]
          }
        }
        n85 = Unbundle By Name(w91) -> ("Yaw"=→"Yaw":dbl, "Fused Heading"=→"Fused Heading":dbl)  [unwired: 3 out]
        n86 = call <vilib>:"Displacement.vi"("NavX Info In"=w86) -> ("Displacement"=→"Displacement":T1, "NavX Info Out"=w85:T25)  [unwired: 9 in]
        n87 = call "FGV Bool.vi"("Init/Read/Write State"=States_for_Action_Engine."Read") -> ("Output node"=w93:bool)  [unwired: 2 in, 1 out]
      }
      n88 = while {
        tunnel: w36 -> [w597]
        tunnel: w35 -> [w594]
        stop <- w591 stop-if-true
        # "Status Loop for Action Queues"
        n89 = Get Queue Status(queue=w597, return elements? (F)=TRUE) -> (error out=w593:errorcluster, # elements in queue=→"Action Queue Items":i32, elements=→"Action Queues items":string[])  [unwired: 1 in, 5 out]
        n90 = Get Queue Status(queue=w594, return elements? (F)=TRUE) -> (# pending remove=→"State Logic Queue Items":i32, error out=w592:errorcluster)  [unwired: 1 in, 6 out]
        n91 = Merge Errors(w593, w592) -> (w591:errorcluster)
        n92 = Wait (ms)(milliseconds to wait=u32 500) -> ()  [unwired: 1 out]
      }
      n93 = while {
        tunnel: w35 -> [w104]
        shift-right: [w115] -> _
        shift-left: TLB_MHL_States."Startup" ("Enum") -> [w109]
        tunnel: w36 -> [w120]
        tunnel: w39 -> [w118]
        tunnel: [w117] -> _
        tunnel: [w116] -> w31
        shift-right: [w106] -> _
        shift-left: T7 {"Front Ultrasonic Obstruct"=TRUE, "Left Ultrasonic Obstruct"=FALSE, "Right Ultrasonic Obstruct "=FALSE} -> [w108]
        stop <- w102 stop-if-true
        # ">>> Motor control cluster >>>"
        # ">>Error  >>"
        # ">>Action states Queue Reference >>"
        # ">>State Logic Queue Reference >>"
        # "TOP LEVEL BASELINE (MAIN PROCESSING LOOP)"
        n94 = Dequeue Element(queue=w120, timeout in ms (-1)=0, error in (no error)=w118) -> (queue out=w110:refnum<queue>, element=w119:string, error out=w111:errorcluster)  [unwired: 1 out]
        "Action State" <- w119
        n95 = Wait Until Next ms Multiple(millisecond multiple=u32 10) -> ()  [unwired: 1 out]
        n96 = case shown="\"Forward\"" w119 {
          tunnel: [w423 w438 w445 w450 w456 w463 w469 w473 w481 w486 w495 w502 TLB_MHL_States."Shutdown" ("Enum") w512 w521 w524 w535 w546 w554 w566 w570] -> w121
          tunnel: [w426 0 0 0 0 0 0 0 0 0 0 0 0 0 0 0 0 0 0 0 0] -> w114
          tunnel: [TRUE FALSE FALSE FALSE FALSE FALSE FALSE FALSE FALSE FALSE FALSE FALSE FALSE FALSE FALSE FALSE FALSE FALSE FALSE FALSE FALSE] -> w113
          tunnel: w110 -> [_ _ _ _ _ _ _ _ _ _ _ _ _ _ _ _ _ _ _ _ _]
          tunnel: w109 -> [w423 w438 w445 w450 w456 w463 w469 w473 w481 w486 w495 w502 _ w512 w521 w524 w535 w546 w554 w566 w570]
          tunnel: w108 -> [w424 w433 w441 w451 w453 w459 w465 w471 w477 w483 w492 w498 w505 w513 w520 w527 w536 w547 w553 w563 w571]
          tunnel: [w424 w432 w440 w451 w453 w459 w465 w471 w477 w483 w491 w498 w505 w513 w517 w526 w536 w547 w553 w563 w571] -> w107
          tunnel: [_ _ _ _ _ _ _ _ _ _ _ _ _ _ _ _ _ w537 w549 w557 _] -> w105
          tunnel: [_ _ _ _ _ _ _ _ _ _ _ _ TRUE _ _ _ _ _ _ _ _] -> w102
          tunnel: [T10."LAST STATE" ("Move mode") T10."INIT" ("Move mode") T10."FORWARD" ("Move mode") T10."LAST STATE" ("Move mode") T10."BACKWARD" ("Move mode") T10."RIGHT" ("Move mode") T10."LEFT" ("Move mode") T10."RCW" ("Move mode") T10."ACW" ("Move mode") T10."STOP" ("Move mode") _ T10."RESET ENCODERS" ("Move mode") T10."INIT" ("Move mode") T10."INIT" ("Move mode") _ _ _ _ _ _ _] -> w100
          frame "No action", Default {
            n97 = case shown="1, Default" w423 {
              tunnel: [0 100] -> w426
              frame 1, Default {
              }
              frame 2 {
              }
            }
            n98 = local write "NavX Zero Yaw"(FALSE ("NavX Zero Yaw")) -> ()
          }
          frame "Init" {
            # ">>State Logic  >>"
            n99 = local write "Servo Angle"(u8 90 ("Servo Angle")) -> ()
            n100 = Bundle By Name(cluster=w433, "Front Ultrasonic Obstruct"=FALSE ("Object detected"), "L IR Sensor"=0.0, "Right Ultrasonic Obstruct"=FALSE ("In move state?")) -> (w432:T7)
          }
          frame "Forward" {
            n101 = local write "NavX Zero Yaw"(FALSE ("NavX Zero Yaw")) -> ()
            n102 = Bundle By Name(cluster=w441, "Right Ultrasonic Obstruct"=TRUE ("In move state?")) -> (w440:T7)
          }
          frame " Motor Control" {
          }
          frame "Reverse" {
            n103 = local write "NavX Zero Yaw"(FALSE ("NavX Zero Yaw")) -> ()
          }
          frame "Right" {
            n104 = local write "NavX Zero Yaw"(FALSE ("NavX Zero Yaw")) -> ()
          }
          frame "Left" {
            n105 = local write "NavX Zero Yaw"(FALSE ("NavX Zero Yaw")) -> ()
          }
          frame "Rotate CW" {
            n106 = local write "NavX Zero Yaw"(FALSE ("NavX Zero Yaw")) -> ()
          }
          frame "Rotate ACW" {
            n107 = local write "NavX Zero Yaw"(FALSE ("NavX Zero Yaw")) -> ()
          }
          frame "Stop" {
            n108 = local write "NavX Zero Yaw"(FALSE ("NavX Zero Yaw")) -> ()
          }
          frame "Software reset" {
            w488 = FALSE ("NavX Zero Yaw")
            n109 = Wait (ms)(milliseconds to wait=u32 20) -> ()  [unwired: 1 out]
            n110 = local write "NavX Zero Yaw"(w488) -> ()
            n111 = Bundle By Name(cluster=w492, "Front Ultrasonic Obstruct"=w488, "L IR Sensor"=0.0, "Right Ultrasonic Obstruct"=w488) -> (w491:T7)
          }
          frame "Hardware reset" {
            n112 = Wait (ms)(milliseconds to wait=u32 100) -> ()  [unwired: 1 out]
            n113 = local write "NavX Zero Yaw"(TRUE ("NavX Zero Yaw")) -> ()
          }
          frame "Exit" {
          }
          frame "Pre-Exit" {
          }
          frame "Ultrasonic read" {
            # "Object detection"
            n114 = local read "L/R average"() -> (w514:fxp<+,64,64>)
            n115 = Less Or Equal?(x=w514, y=35.0) -> (x <= y?=w515:bool)
            n116 = Bundle By Name(cluster=w520, "Front Ultrasonic Obstruct"=w515) -> (w517:T7)
          }
          frame "IR Sensor Read" {
            n117 = local read "Left IR Sensor"() -> (w525:dbl)
            n118 = Bundle By Name(cluster=w527, "L IR Sensor"=w525) -> (w526:T7)
          }
          frame "Calculate" {
            n119 = Unbundle By Name(w536) -> ("L IR Sensor"=w531:dbl)
            n120 = call-poly <vilib>:"PID.vi"("output range"=cluster{"output high":dbl, "output low":dbl} {"output high"=0.3, "output low"=-0.3}, "PID gains"=T11 {"proportional gain (Kc)"=0.01, "integral time (Ti, min)"=0.0, "derivative time (Td, min)"=0.0}, "process variable"=w531, "setpoint"=20.0) -> ("output"=w528:dbl)  [unwired: 6 in, 1 out]
            n121 = Negate(x=w528) -> ()  [unwired: 1 out]
          }
          frame "Cam Init" {
            n122 = call "Low-Level Grab.vi"("States"=State_control."Initialise", "Session In"=T13 "cam1") -> ("error out"=w538:errorcluster, "Session Out"=w539:T13)  [unwired: 7 in, 1 out]
            n123 = call "Low-Level Grab.vi"("error in (no error)"=w538, "States"=State_control."Start camera", "Session In"=w539) -> ("error out"=w537:errorcluster)  [unwired: 6 in, 2 out]
            n124 = local write "Servo Angle"(u8 170 ("Servo Angle")) -> ()
          }
          frame "Cam Acq" {
            n125 = call "Low-Level Grab.vi"("States"=State_control."Continuous Acquisition ") -> ("error out"=w550:errorcluster, "Image Out"=w551:T27)  [unwired: 8 in, 1 out]
            n126 = call "All object detection ver2.vi"("Image In"=w551, "error in"=w550) -> ("Object detection count"=→"Object detection count":T2, "error out"=w549:errorcluster)  [unwired: 1 out]
          }
          frame "Cam Exit" {
            n127 = call "Low-Level Grab.vi"("States"=State_control."Stop camera") -> ("error out"=w558:errorcluster, "Session Out"=w560:T13)  [unwired: 8 in, 1 out]
            n128 = local write "Servo Angle"(u8 90 ("Servo Angle")) -> ()
            n129 = call "Low-Level Grab.vi"("error in (no error)"=w558, "States"=State_control."Dispose all", "Session In"=w560) -> ("error out"=w557:errorcluster)  [unwired: 6 in, 2 out]
          }
          frame "NavX Calibrate" {
            # "Adds a 15 second delay to the startup process \nfor the NavX to calibrate"
            n130 = Wait (ms)(milliseconds to wait=u32 15000) -> ()  [unwired: 1 out]
          }
        }
        "State logic" <- w121
        "Camera error" <- w105
        n131 = local read "Yaw"() -> (w98:dbl)
        n132 = call "New motor Control integrated remodeled state based.vi"("Yaw"=w98, "States"=w100) -> ("Speed and distance cluster"=w99:T28)  [unwired: 1 in, 1 out]
        n133 = case shown="True" w113 {
          tunnel: w121 -> [w125 w135]
          tunnel: w104 -> [w126 w134]
          tunnel: w110 -> [w124 w130]
          tunnel: [w126 w134] -> w117
          tunnel: [w124 w146] -> w116
          tunnel: [w125 w145] -> w115
          tunnel: w111 -> [_ w144]
          tunnel: w114 -> [_ w143]
          tunnel: w107 -> [w123 w137]
          tunnel: [w123 w137] -> w106
          tunnel: [enum16{"OFF", "ON", "BLINK"}."BLINK" ("GREEN LED State") w131] -> w101
          tunnel: w99 -> [_ w128]
          frame False {
          }
          frame True {
            # ">>State Logic Queue Reference >>"
            n134 = Get Queue Status(queue=w134) -> (error out=w133:errorcluster)  [unwired: 2 in, 7 out]
            n135 = local read "DIO 1"() -> (w132:bool)
            n136 = Unbundle(w128) -> (w127:T29)  [unwired: 1 out]
            n137 = case shown="No Error" w133 {
              tunnel: [w147 TLB_MHL_States."Reset" ("Enum")] -> w136
              tunnel: w135 -> [w147 _]
              frame No Error {
              }
              frame Error {
              }
            }
            n138 = Unbundle By Name(w137) -> ("Front Ultrasonic Obstruct"=w138:bool, "Right Ultrasonic Obstruct"=w129:bool)  [unwired: 1 out]
            n139 = local read "Fused Heading"() -> (w139:dbl)
            n140 = Unbundle By Name(w127) -> ("xDistance"=w140:dbl, "yDistance"=w142:dbl, "wDistance"=w141:dbl)
            n141 = case shown="20" w136 {
              tunnel: w134 -> [w152 w217 w228 w245 w264 w280 w295 w311 w327 w343 _ w367 w384 w396 _ _ _]
              tunnel: w130 -> [_ w220 w234 w249 w273 w284 w300 w317 w332 w349 w360 w370 w385 w400 w409 w413 w419]
              tunnel: [w149 w219 w233 w250 w272 w285 w299 w316 w331 w348 w359 w371 w386 w399 w409 w412 w419] -> w146
              tunnel: [w155 TLB_MHL_States."Idle" ("Enum") w236 w251 w269 w288 w302 w315 w333 w347 TLB_MHL_States."Shutdown" ("Enum") w373 w387 w398 TLB_MHL_States."Reset" ("Enum") TLB_MHL_States."Shutdown" ("Enum") TLB_MHL_States."Reset" ("Enum")] -> w145
              tunnel: w144 -> [w153 _ _ _ _ _ _ _ _ _ _ _ _ _ _ _ _]
              tunnel: w143 -> [w154 _ _ _ _ _ _ _ _ _ _ _ _ _ _ _ _]
              tunnel: w132 -> [_ _ w231 w248 w267 _ _ _ _ w346 _ w368 w382 w397 _ _ _]
              tunnel: w142 -> [_ _ w226 _ _ _ w294 w310 _ _ _ _ _ _ _ _ _]
              tunnel: w141 -> [_ _ _ _ _ _ _ _ _ _ _ _ _ _ _ _ _]
              tunnel: w140 -> [_ _ _ _ _ _ _ _ w326 _ _ _ _ _ _ _ _]
              tunnel: w139 -> [_ _ _ _ w263 _ _ _ _ _ _ _ _ _ _ _ _]
              tunnel: w138 -> [_ _ _ w246 _ w282 _ _ _ w345 _ _ _ _ _ _ _]
              tunnel: [enum16{"OFF", "ON", "BLINK"}."ON" ("GREEN LED State") enum16{"OFF", "ON", "BLINK"}."OFF" ("GREEN LED State") enum16{"OFF", "ON", "BLINK"}."BLINK" ("GREEN LED State") enum16{"OFF", "ON", "BLINK"}."BLINK" ("GREEN LED State") enum16{"OFF", "ON", "BLINK"}."BLINK" ("GREEN LED State") enum16{"OFF", "ON", "BLINK"}."BLINK" ("GREEN LED State") enum16{"OFF", "ON", "BLINK"}."BLINK" ("GREEN LED State") enum16{"OFF", "ON", "BLINK"}."BLINK" ("GREEN LED State") enum16{"OFF", "ON", "BLINK"}."BLINK" ("GREEN LED State") enum16{"OFF", "ON", "BLINK"}."BLINK" ("GREEN LED State") enum16{"OFF", "ON", "BLINK"}."OFF" ("GREEN LED State") enum16{"OFF", "ON", "BLINK"}."BLINK" ("GREEN LED State") enum16{"OFF", "ON", "BLINK"}."BLINK" ("GREEN LED State") enum16{"OFF", "ON", "BLINK"}."BLINK" ("GREEN LED State") _ enum16{"OFF", "ON", "BLINK"}."OFF" ("GREEN LED State") _] -> w131
              tunnel: w130 -> [w150 _ _ _ _ _ _ _ _ _ _ _ _ _ _ _ _]
              tunnel: w129 -> [_ _ _ _ _ _ _ _ _ _ _ _ w380 _ _ _ _]
              frame 2, Default {
                # ">>State Logic >>"
                n142 = Dequeue Element(queue=w152, timeout in ms (-1)=w154, error in (no error)=w153) -> (element=w156:T3)  [unwired: 3 out]
                "element" <- w156
                n143 = case shown="\"Start Drive Straight\"" w156 {
                  tunnel: [TLB_MHL_States."Idle" ("Enum") TLB_MHL_States."Idle" ("Enum") TLB_MHL_States."Task 1" ("Enum") TLB_MHL_States."Task 2" ("Enum") TLB_MHL_States."Task 3" ("Enum") TLB_MHL_States."Task 4" ("Enum") TLB_MHL_States."Shutdown" ("Enum") TLB_MHL_States."Wall follow mode" ("Enum") TLB_MHL_States."Acquire image" ("Enum") TLB_MHL_States."Drive Straight" ("Enum")] -> w155
                  tunnel: w150 -> [w157 w159 w163 w170 w176 w184 w191 w198 w205 w212]
                  tunnel: [w157 w159 w162 w169 w177 w183 w190 w197 w204 w210] -> w149
                  frame "Start Sequence" {
                    # "This event should never be triggered"
                  }
                  frame "Idle", Default {
                    # ">>Action states Queue Reference >>"
                  }
                  frame "Start Task 1" {
                    # ">>Action states Queue Reference >>"
                    # "Action items"
                    n144 = for {
                      shift-right: [w167] -> w162
                      shift-left: w163 -> [w166]
                      tunnel: string[] ["Hardware reset", "Software reset", "Forward", ""] -> [w165] mode=indexing
                      n145 = Enqueue Element(queue=w166, element=w165) -> (queue out=w167:refnum<queue>)  [unwired: 2 in, 2 out]
                    }
                  }
                  frame "Start Task 2" {
                    # ">>Action states Queue Reference >>"
                    # "Action items"
                    n146 = for {
                      shift-right: [w174] -> w169
                      shift-left: w170 -> [w173]
                      tunnel: string[] ["Hardware reset", "Software reset", ""] -> [w172] mode=indexing
                      n147 = Enqueue Element(queue=w173, element=w172) -> (queue out=w174:refnum<queue>)  [unwired: 2 in, 2 out]
                    }
                  }
                  frame "Start Task 3" {
                    # ">>Action states Queue Reference >>"
                    n148 = for {
                      shift-right: [w181] -> w177
                      shift-left: w176 -> [w180]
                      tunnel: string[] ["Hardware reset", "Software reset", ""] -> [w179] mode=indexing
                      n149 = Enqueue Element(queue=w180, element=w179) -> (queue out=w181:refnum<queue>)  [unwired: 2 in, 2 out]
                    }
                  }
                  frame "Start Task 4" {
                    # ">>Action states Queue Reference >>"
                    # "Action items"
                    n150 = for {
                      shift-right: [w188] -> w183
                      shift-left: w184 -> [w187]
                      tunnel: string[] ["Hardware reset", "Software reset", ""] -> [w186] mode=indexing
                      n151 = Enqueue Element(queue=w187, element=w186) -> (queue out=w188:refnum<queue>)  [unwired: 2 in, 2 out]
                    }
                  }
                  frame "Exit" {
                    # ">>Action states Queue Reference >>"
                    # "Action items"
                    n152 = for {
                      shift-right: [w195] -> w190
                      shift-left: w191 -> [w194]
                      tunnel: string[] ["Hardware reset", "Software reset", "Motor Control", "Pre-Exit", "Exit"] -> [w193] mode=indexing
                      n153 = Enqueue Element(queue=w194, element=w193) -> (queue out=w195:refnum<queue>)  [unwired: 2 in, 2 out]
                    }
                  }
                  frame "Wall follow mode" {
                    # ">>Action states Queue Reference >>"
                    # "Action items"
                    n154 = for {
                      shift-right: [w202] -> w197
                      shift-left: w198 -> [w201]
                      tunnel: string[] ["Hardware reset", "Software reset", ""] -> [w200] mode=indexing
                      n155 = Enqueue Element(queue=w201, element=w200) -> (queue out=w202:refnum<queue>)  [unwired: 2 in, 2 out]
                    }
                  }
                  frame "Camera vision" {
                    # ">>Action states Queue Reference >>"
                    # "Action items"
                    n156 = for {
                      shift-right: [w209] -> w204
                      shift-left: w205 -> [w208]
                      tunnel: string[] ["Hardware reset", "Software reset", "Cam Init", "Cam Acq"] -> [w207] mode=indexing
                      n157 = Enqueue Element(queue=w208, element=w207) -> (queue out=w209:refnum<queue>)  [unwired: 2 in, 2 out]
                    }
                  }
                  frame "Start Drive Straight" {
                    # ">>Action states Queue Reference >>"
                    # "Action items"
                    n158 = for {
                      shift-right: [w216] -> w210
                      shift-left: w212 -> [w215]
                      tunnel: string[] ["Hardware reset", "Software reset", "Forward", ""] -> [w214] mode=indexing
                      n159 = Enqueue Element(queue=w215, element=w214) -> (queue out=w216:refnum<queue>)  [unwired: 2 in, 2 out]
                    }
                  }
                }
              }
              frame 1 {
                # ">>State Logic >>"
                n160 = Flush Queue(queue=w217) -> ()  [unwired: 1 in, 3 out]
                n161 = for {
                  shift-right: [w224] -> w219
                  shift-left: w220 -> [w225]
                  tunnel: string[] ["Init", "NavX Calibrate", "Software reset", "Hardware reset", "Motor Control"] -> [w223] mode=indexing
                  n162 = Enqueue Element(queue=w225, element=w223) -> (queue out=w224:refnum<queue>)  [unwired: 2 in, 2 out]
                }
              }
              frame 6 {
                # ">>State Logic >>"
                n163 = Greater Or Equal?(x=w226, y=1.0) -> (x >= y?=w229:bool)
                n164 = Or(x=w231, y=w229) -> (x .or. y?=w232:bool)
                n165 = case shown="True" w232 {
                  tunnel: [string[] ["Forward", "Motor Control", ""] string[] ["Software reset", "Hardware reset", "Motor Control"]] -> w235
                  frame False {
                  }
                  frame True {
                  }
                }
                n166 = Flush Queue(queue=w228) -> ()  [unwired: 1 in, 3 out]
                n167 = Select(t=TLB_MHL_States."Idle" ("Enum"), s=w232, f=TLB_MHL_States."Task 1" ("Enum")) -> (s? t:f=w236:T4)
                n168 = for {
                  shift-right: [w242] -> w233
                  shift-left: w234 -> [w243]
                  tunnel: w235 -> [w241] mode=indexing
                  n169 = Enqueue Element(queue=w243, element=w241) -> (queue out=w242:refnum<queue>)  [unwired: 2 in, 2 out]
                }
              }
              frame 7 {
                # ">>State Logic >>"
                n170 = Flush Queue(queue=w245) -> ()  [unwired: 1 in, 3 out]
                n171 = case shown="True" w248 {
                  tunnel: [w255 string[] ["Hardware reset", "Software reset", "Motor control"]] -> w247
                  tunnel: w246 -> [w254 _]
                  frame False {
                    n172 = case shown="False" w254 {
                      tunnel: [string[] ["Stop", "Ultrasonic read", "Motor Control"] string[] ["Reverse", "Ultrasonic read", "Motor control"]] -> w255
                      frame False {
                      }
                      frame True {
                      }
                    }
                  }
                  frame True {
                  }
                }
                n173 = Select(t=TLB_MHL_States."Idle" ("Enum"), s=w248, f=TLB_MHL_States."Task 2" ("Enum")) -> (s? t:f=w251:T4)
                n174 = for {
                  shift-right: [w260] -> w250
                  shift-left: w249 -> [w261]
                  tunnel: w247 -> [w259] mode=indexing
                  n175 = Enqueue Element(queue=w261, element=w259) -> (queue out=w260:refnum<queue>)  [unwired: 2 in, 2 out]
                }
              }
              frame 8 {
                n176 = Greater Or Equal?(x=w263, y=360.0) -> (x >= y?=w266:bool)
                n177 = Flush Queue(queue=w264) -> ()  [unwired: 1 in, 3 out]
                n178 = Or(x=w266, y=w267) -> (x .or. y?=w268:bool)
                n179 = case shown="False" w268 {
                  tunnel: [string[] ["Rotate CW", "Motor Control"] string[] ["Software reset", "Hardware reset", "Motor Control"]] -> w274
                  frame False {
                  }
                  frame True {
                  }
                }
                n180 = for {
                  shift-right: [w276] -> w272
                  shift-left: w273 -> [w277]
                  tunnel: w274 -> [w275] mode=indexing
                  n181 = Enqueue Element(queue=w277, element=w275) -> (queue out=w276:refnum<queue>)  [unwired: 2 in, 2 out]
                }
                n182 = Select(t=TLB_MHL_States."Idle" ("Enum"), s=w268, f=TLB_MHL_States."Task 3" ("Enum")) -> (s? t:f=w269:T4)
              }
              frame 9 {
                n183 = Flush Queue(queue=w280) -> ()  [unwired: 1 in, 3 out]
                n184 = case shown="True" w282 {
                  tunnel: [string[] ["Forward", "Ultrasonic read", "Motor Control"] string[] ["Stop", "Hardware reset", "Software reset", "Motor Control"]] -> w283
                  frame False {
                  }
                  frame True {
                  }
                }
                n185 = for {
                  shift-right: [w292] -> w285
                  shift-left: w284 -> [w293]
                  tunnel: w283 -> [w291] mode=indexing
                  n186 = Enqueue Element(queue=w293, element=w291) -> (queue out=w292:refnum<queue>)  [unwired: 2 in, 2 out]
                }
                n187 = Select(t=TLB_MHL_States."Task 4a" ("Enum"), s=w282, f=TLB_MHL_States."Task 4" ("Enum")) -> (s? t:f=w288:T4)
              }
              frame 10 {
                n188 = Greater Or Equal?(x=w294, y=0.5) -> (x >= y?=w298:bool)
                n189 = Flush Queue(queue=w295) -> ()  [unwired: 1 in, 3 out]
                n190 = case shown="True" w298 {
                  tunnel: [string[] ["Right", "Motor Control"] string[] ["Stop", "Hardware reset", "Software reset", "Motor Control"]] -> w301
                  frame False {
                  }
                  frame True {
                  }
                }
                n191 = for {
                  shift-right: [w308] -> w299
                  shift-left: w300 -> [w309]
                  tunnel: w301 -> [w307] mode=indexing
                  n192 = Enqueue Element(queue=w309, element=w307) -> (queue out=w308:refnum<queue>)  [unwired: 2 in, 2 out]
                }
                n193 = Select(t=TLB_MHL_States."Task 4b" ("Enum"), s=w298, f=TLB_MHL_States."Task 4a" ("Enum")) -> (s? t:f=w302:T4)
              }
              frame 11 {
                n194 = Flush Queue(queue=w311) -> ()  [unwired: 1 in, 3 out]
                n195 = Greater Or Equal?(x=w310, y=0.75) -> (x >= y?=w313:bool)
                n196 = case shown="False" w313 {
                  tunnel: [string[] ["Forward", "Motor control"] string[] ["Stop", "Hardware reset", "Software reset"]] -> w318
                  frame False {
                  }
                  frame True {
                  }
                }
                n197 = for {
                  shift-right: [w324] -> w316
                  shift-left: w317 -> [w325]
                  tunnel: w318 -> [w323] mode=indexing
                  n198 = Enqueue Element(queue=w325, element=w323) -> (queue out=w324:refnum<queue>)  [unwired: 2 in, 2 out]
                }
                n199 = Select(t=TLB_MHL_States."Task 4c" ("Enum"), s=w313, f=TLB_MHL_States."Task 4b" ("Enum")) -> (s? t:f=w315:T4)
              }
              frame 12 {
                n200 = Flush Queue(queue=w327) -> ()  [unwired: 1 in, 3 out]
                n201 = Less Or Equal?(x=w326, y=-0.65) -> (x <= y?=w329:bool)
                n202 = case shown="False" w329 {
                  tunnel: [string[] ["Left", "Motor Control"] string[] ["Stop", "Hardware reset", "Software reset", "Motor Control"]] -> w334
                  frame False {
                  }
                  frame True {
                  }
                }
                n203 = for {
                  shift-right: [w340] -> w331
                  shift-left: w332 -> [w341]
                  tunnel: w334 -> [w339] mode=indexing
                  n204 = Enqueue Element(queue=w341, element=w339) -> (queue out=w340:refnum<queue>)  [unwired: 2 in, 2 out]
                }
                n205 = Select(t=TLB_MHL_States."Task 4d" ("Enum"), s=w329, f=TLB_MHL_States."Task 4c" ("Enum")) -> (s? t:f=w333:T4)
              }
              frame 13 {
                n206 = Flush Queue(queue=w343) -> ()  [unwired: 1 in, 3 out]
                n207 = Or(x=w346, y=w345) -> (x .or. y?=w344:bool)
                n208 = case shown="True" w344 {
                  tunnel: [string[] ["Forward", "Ultrasonic Read", "Motor Control"] string[] ["Stop", "Hardware reset", "Software reset", "Motor Control"]] -> w350
                  frame False {
                  }
                  frame True {
                  }
                }
                n209 = for {
                  shift-right: [w356] -> w348
                  shift-left: w349 -> [w357]
                  tunnel: w350 -> [w355] mode=indexing
                  n210 = Enqueue Element(queue=w357, element=w355) -> (queue out=w356:refnum<queue>)  [unwired: 2 in, 2 out]
                }
                n211 = Select(t=TLB_MHL_States."Idle" ("Enum"), s=w344, f=TLB_MHL_States."Task 4d" ("Enum")) -> (s? t:f=w347:T4)
              }
              frame 5 {
                n212 = for {
                  shift-right: [w364] -> w359
                  shift-left: w360 -> [w365]
                  tunnel: string[] ["Software reset", "Hardware reset", "Motor Control"] -> [w363] mode=indexing
                  n213 = Enqueue Element(queue=w365, element=w363) -> (queue out=w364:refnum<queue>)  [unwired: 2 in, 2 out]
                }
              }
              frame 19 {
                n214 = Flush Queue(queue=w367) -> ()  [unwired: 1 in, 3 out]
                n215 = case shown="False" w368 {
                  tunnel: [string[] ["IR Sensor Read", "Calculate", "Forward", "Motor Control"] string[] ["Hardware reset", "Software reset", "Motor Control"]] -> w369
                  frame False {
                  }
                  frame True {
                  }
                }
                n216 = for {
                  shift-right: [w378] -> w371
                  shift-left: w370 -> [w379]
                  tunnel: w369 -> [w377] mode=indexing
                  n217 = Enqueue Element(queue=w379, element=w377) -> (queue out=w378:refnum<queue>)  [unwired: 2 in, 2 out]
                }
                n218 = Select(t=TLB_MHL_States."Idle" ("Enum"), s=w368, f=TLB_MHL_States."Wall follow mode" ("Enum")) -> (s? t:f=w373:T4)
              }
              frame 20 {
                n219 = Flush Queue(queue=w384) -> ()  [unwired: 1 in, 3 out]
                n220 = case shown="False" w382 {
                  tunnel: [string[] ["Forward"] string[] ["Hardware reset", "Software reset", "Motor Control", ""]] -> w381
                  tunnel: w380 -> [_ _]
                  frame False {
                  }
                  frame True {
                  }
                }
                n221 = for {
                  shift-right: [w393] -> w386
                  shift-left: w385 -> [w394]
                  tunnel: w381 -> [w392] mode=indexing
                  n222 = Enqueue Element(queue=w394, element=w392) -> (queue out=w393:refnum<queue>)  [unwired: 2 in, 2 out]
                }
                n223 = Select(t=TLB_MHL_States."Idle" ("Enum"), s=w382, f=TLB_MHL_States."Drive Straight" ("Enum")) -> (s? t:f=w387:u16)
              }
              frame 18 {
                n224 = Flush Queue(queue=w396) -> ()  [unwired: 1 in, 3 out]
                n225 = case shown="True" w397 {
                  tunnel: [string[] ["Cam Acq"] string[] ["Hardware reset", "Software reset", "Cam Exit", ""]] -> w401
                  frame False {
                  }
                  frame True {
                  }
                }
                n226 = for {
                  shift-right: [w407] -> w399
                  shift-left: w400 -> [w408]
                  tunnel: w401 -> [w406] mode=indexing
                  n227 = Enqueue Element(queue=w408, element=w406) -> (queue out=w407:refnum<queue>)  [unwired: 2 in, 2 out]
                }
                n228 = Select(t=TLB_MHL_States."Idle" ("Enum"), s=w397, f=TLB_MHL_States."Acquire image" ("Enum")) -> (s? t:f=w398:T4)
              }
              frame 3 {
              }
              frame 4 {
                # ">>State Logic >>"
                n229 = for {
                  shift-right: [w417] -> w412
                  shift-left: w413 -> [w418]
                  tunnel: string[] ["Software reset", "Hardware reset", "Motor Control", "Cam Exit", "Pre-Exit", "Exit"] -> [w416] mode=indexing
                  n230 = Enqueue Element(queue=w418, element=w416) -> (queue out=w417:refnum<queue>)  [unwired: 2 in, 2 out]
                }
              }
              frame 0 {
              }
            }
          }
        }
        n231 = local write "GREEN LED State"(w101) -> ()
      }
      n232 = call <vilib>:"NavX Close.vi"("NavX Info In"=w28) -> ()  [unwired: 10 in, 1 out]
      n233 = while {
        shift-right: [w62] -> _
        shift-left: _ -> [w63]
        shift-right: [w61] -> _
        shift-left: _ -> [w60]
        stop <- w69 stop-if-true
        (unwired) TRUE
        # "LED Blinker Loop"
        n234 = case shown="\"BLINK\"" "GREEN LED State" {
          tunnel: [FALSE TRUE w77] -> w65
          tunnel: w63 -> [_ _ w77]
          tunnel: [_ _ w78] -> w62
          frame "OFF", Default {
          }
          frame "ON" {
          }
          frame "BLINK" {
            n235 = Not(x=w77) -> (.not. x?=w78:bool)
          }
        }
        n236 = case shown="\"OFF\", Default" "RED LED State" {
          tunnel: [FALSE TRUE w73] -> w64
          tunnel: [_ _ w74] -> w61
          tunnel: w60 -> [_ _ w73]
          frame "OFF", Default {
          }
          frame "ON" {
          }
          frame "BLINK" {
            n237 = Not(x=w73) -> (.not. x?=w74:bool)
          }
        }
        n238 = local write "Green LED"(w65) -> ()
        n239 = local write "Red LED"(w64) -> ()
        n240 = call "FGV Bool.vi"("Init/Read/Write State"=States_for_Action_Engine."Read") -> ("Output node"=w69:bool)  [unwired: 2 in, 1 out]
        n241 = Wait (ms)(milliseconds to wait=u32 500) -> ()  [unwired: 1 out]
      }
      n242 = call <vilib>:"DIO Close.vi"("DIO Info In"=w3) -> ()  [unwired: 10 in, 1 out]
      n243 = call <vilib>:"DIO Close.vi"("error in (no error)"=w20, "DIO Info In"=w26) -> ()  [unwired: 9 in, 1 out]
      n244 = call <vilib>:"DIO Close.vi"("error in (no error)"=w18, "DIO Info In"=w22) -> ()  [unwired: 9 in, 1 out]
      n245 = call <vilib>:"DIO Close.vi"("error in (no error)"=w8, "DIO Info In"=w13) -> ()  [unwired: 9 in, 1 out]
      n246 = call <vilib>:"DIO Close.vi"("error in (no error)"=w6, "DIO Info In"=w12) -> ()  [unwired: 9 in, 1 out]
      n247 = Merge Errors "Merge Errors"(w53, w52) -> (w34:errorcluster)
      n248 = Merge Errors(w38, w34) -> (w29:errorcluster)
      n249 = Destroy User Event(user event=w56, error in=w29) -> ()  [unwired: 1 out]
      n250 = Destroy User Event(user event=w57, error in=w29) -> ()  [unwired: 1 out]
      n251 = Unregister For Events(event registration refnum=w48, error in=w29) -> ()  [unwired: 1 out]
      n252 = Release Queue(queue=w31, error in (no error)=w29) -> (error out=→"error out":errorcluster)  [unwired: 1 in, 2 out]
      n253 = Release Queue(queue=w47, error in (no error)=w29) -> ()  [unwired: 1 in, 3 out]
    }
    frame #2 {
      (unwired) T15."INIT" ("States")
      n254 = call "New motor Control integrated remodeled state based.vi"() -> ()  [unwired: 3 in, 2 out]
    }
    frame #3 {
    }
  }
